vi "test Scheduled Loopback with Disable.vi"(8 "error in":errorcluster, 11 "TestCase in":refnum<class "Single Board Loopback.lvclass">) -> (0 "error out":errorcluster, 3 "TestCase out":refnum<class "Single Board Loopback.lvclass">)   [LabVIEW 2020, in "Single Board Loopback.lvclass"]
uses:
  Single Board Loopback.lvclass
  <vilib>/addons/_JKI Toolkits/VI Tester/TestCase.llb/TestCase.lvclass
  <vilib>/NI/VeriStand Custom Device Testing Tools/VeriStandTestUtilities/VeriStandTestUtilities.lvlib
  <vilib>/NI VeriStand/Execution/Workspace/NI_VS Workspace ExecutionAPI.lvlib
  <vilib>/NI VeriStand/Execution/Workspace/NI VeriStand - Set Multiple Channel Values.vi
  <vilib>/numeric/Random Number (Range) U64.vi
  C:/Program Files (x86)/National Instruments/LabVIEW 2020/vi.lib/addons/_JKI Toolkits/VI Tester/TestCase.llb/TestCase.lvclass
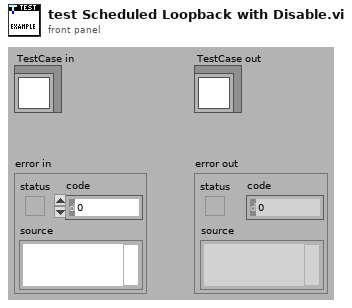
[diagram p1: front panel]
types:
  T1 = typedef "NI_VS Workspace ExecutionAPI.lvlib/WorkspaceAPI.ctl" = refnum<k24>
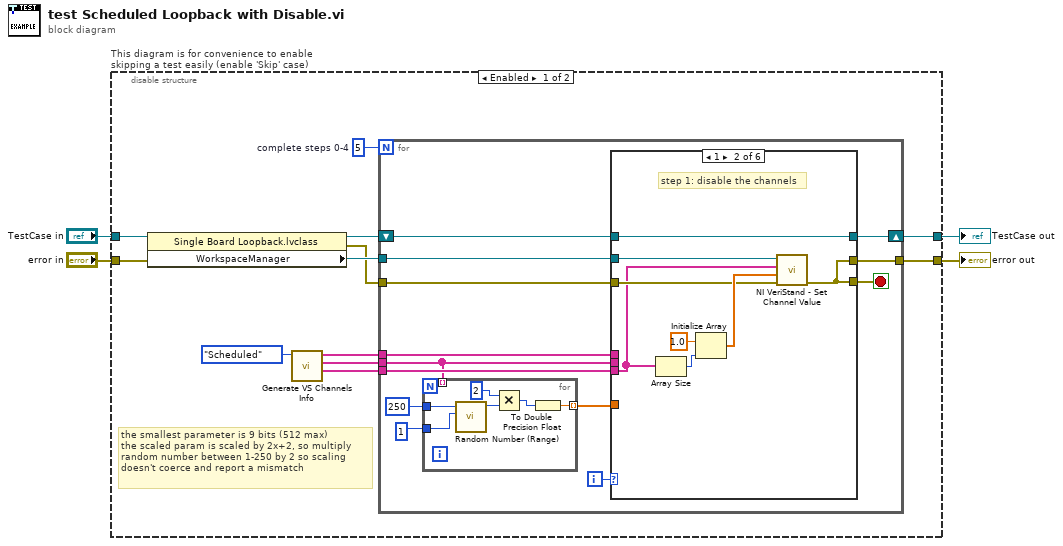
[diagram p0: block diagram]
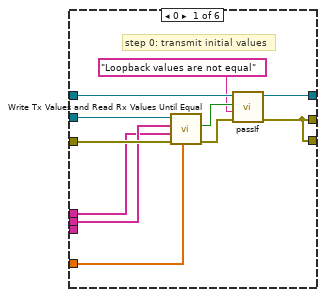
[diagram p2: hidden frame]
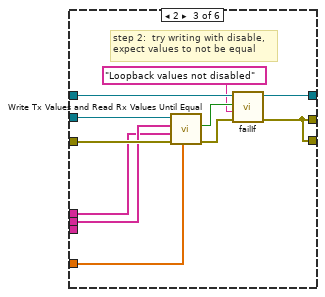
[diagram p3: hidden frame]
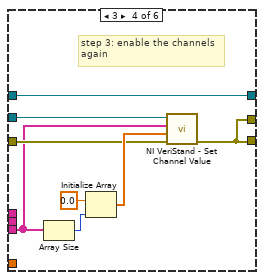
[diagram p4: hidden frame]
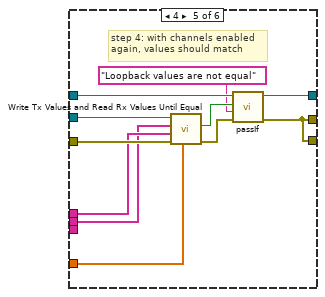
[diagram p5: hidden frame]
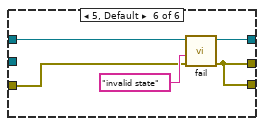
[diagram p6: hidden frame]
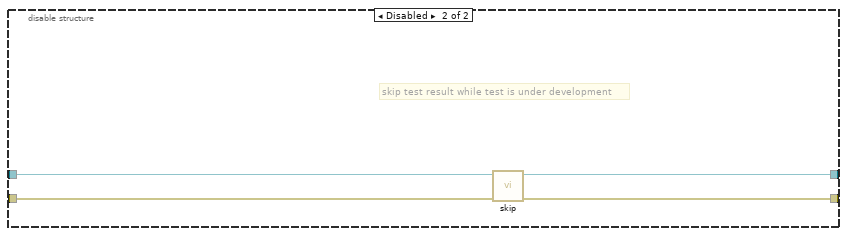
[diagram p7: hidden frame]
diagram:
  n1 = disable-structure "This diagram is for convenience to enable skipping a test easily (enable 'Skip' case)" shown="Enabled" {
    disable-tunnel: "TestCase in" -> [w12 w93]
    disable-tunnel: [w10 w91] -> w1
    disable-tunnel: [w9 w92] -> w3
    disable-tunnel: "error in" -> [w11 w90]
    frame Enabled {
      w6 = 5  # complete steps 0-4
      # "the smallest parameter is 9 bits (512 max)\nthe scaled param is scaled by 2x+2, so multiply \nrandom number between 1-250 by 2 so scaling\ndoesn't coerce and report a mismatch"
      n2 = property class="Single Board Loopback.lvclass"(reference=w12, error in=w11) -> (reference out=w13:refnum<class "Single Board Loopback.lvclass">, error out=w14:errorcluster, "WorkspaceManager"=w15:T1)
      n3 = call "Generate VS Channels Info.vi"("Transfer Type"=enum16{"Acyclic", "Scheduled"}."Scheduled") -> ("Tx Disable Channels Array"=w7:string[], "Tx Channels Array"=w8:string[], "Rx Channels Array"=w16:string[])  [unwired: 6 in, 2 out]
      n4 = for {
        N: w6 -> [_]
        tunnel: w16 -> [w29]
        tunnel: w15 -> [w28]
        tunnel: w14 -> [w27]
        tunnel: w8 -> [w17]
        shift-right: [w25] -> w10
        shift-left: w13 -> [w26]
        tunnel: [w24] -> w9
        tunnel: w7 -> [w21]
        i -> [w23]
        stop <- w22 stop-if-true
        n5 = for {
          tunnel: [w34] -> w20 mode=indexing
          tunnel: u64 250 ("upper bound (100)") -> [w33]
          tunnel: u64 1 ("upper bound (100)") -> [w32]
          tunnel: w17 -> [_] mode=indexing
          n6 = call-poly <vilib>:"Random Number (Range).vi"("lower bound (0)"=w32, "upper bound (100)"=w33) -> ("number"=w35:u64)  [unwired: 9 in]
          n7 = Multiply(x=u64 2, y=w35) -> (x*y=w31:u64)
          n8 = To Double Precision Float(number=w31) -> (double precision float=w34:dbl)
        }
        n9 = case shown="1" w23 {
          tunnel: w29 -> [w37 _ w56 _ w76 _]
          tunnel: w28 -> [w46 w50 w65 w69 w84 _]
          tunnel: w27 -> [w45 w49 w64 w68 w83 w86]
          tunnel: w26 -> [w43 w54 w62 w73 w81 w88]
          tunnel: [w42 w54 w61 w73 w80 w89] -> w25
          tunnel: [w39 w48 w58 w67 w77 w85] -> w24
          tunnel: w17 -> [w38 _ w57 _ w75 _]
          tunnel: [w39 w48 w58 w67 w77 w85] -> w22
          tunnel: w21 -> [_ w47 _ w66 _ _]
          tunnel: w20 -> [w36 _ w55 _ w74 _]
          frame 0 {
            # "step 0: transmit initial values"
            n10 = call <vilib>:"Write Tx Values and Read Rx Values Until Equal.vi"("Tx values"=w36, "error in"=w45, "Rx aliases"=w37, "Tx aliases"=w38, "workspace manager in"=w46) -> ("error out"=w44:errorcluster, "values equal"=w41:bool)  [unwired: 4 in, 1 out]
            n11 = call-dynamic "passIf.vi"("error in (no error)"=w44, "message (\"\")"="Loopback values are not equal" ("message (\"\")"), "pass"=w41, "TestCase in"=w43) -> ("error out"=w39:errorcluster, "TestCase out"=w42:refnum<class "Single Board Loopback.lvclass">)  [unwired: 6 in]
          }
          frame 1 {
            # "step 1: disable the channels"
            n12 = Array Size(array=w47) -> (size(s)=w53:i32)
            n13 = Initialize Array(1.0 ("element"), w53) -> (w51:dbl[])
            n14 = call-poly <vilib>:"NI VeriStand - Set Channel Value.vi"("error in (no error)"=w49, "Values"=w51, "Channels"=w47, "WorkspaceManager in"=w50) -> ("error out"=w48:errorcluster)  [unwired: 6 in, 1 out]
          }
          frame 2 {
            # "step 2:  try writing with disable,\nexpect values to not be equal"
            n15 = call <vilib>:"Write Tx Values and Read Rx Values Until Equal.vi"("Tx values"=w55, "error in"=w64, "Rx aliases"=w56, "Tx aliases"=w57, "workspace manager in"=w65) -> ("error out"=w63:errorcluster, "values equal"=w60:bool)  [unwired: 4 in, 1 out]
            n16 = call-dynamic "failIf.vi"("error in (no error)"=w63, "message (\"\")"="Loopback values not disabled" ("message (\"\")"), "fail"=w60, "TestCase in"=w62) -> ("error out"=w58:errorcluster, "TestCase out"=w61:refnum<class "Single Board Loopback.lvclass">)  [unwired: 6 in]
          }
          frame 3 {
            # "step 3: enable the channels\nagain"
            n17 = Array Size(array=w66) -> (size(s)=w72:i32)
            n18 = Initialize Array(0.0 ("element"), w72) -> (w70:dbl[])
            n19 = call-poly <vilib>:"NI VeriStand - Set Channel Value.vi"("error in (no error)"=w68, "Values"=w70, "Channels"=w66, "WorkspaceManager in"=w69) -> ("error out"=w67:errorcluster)  [unwired: 6 in, 1 out]
          }
          frame 4 {
            # "step 4: with channels enabled\nagain, values should match"
            n20 = call <vilib>:"Write Tx Values and Read Rx Values Until Equal.vi"("Tx values"=w74, "error in"=w83, "Rx aliases"=w76, "Tx aliases"=w75, "workspace manager in"=w84) -> ("error out"=w82:errorcluster, "values equal"=w79:bool)  [unwired: 4 in, 1 out]
            n21 = call-dynamic "passIf.vi"("error in (no error)"=w82, "message (\"\")"="Loopback values are not equal" ("message (\"\")"), "pass"=w79, "TestCase in"=w81) -> ("error out"=w77:errorcluster, "TestCase out"=w80:refnum<class "Single Board Loopback.lvclass">)  [unwired: 6 in]
          }
          frame 5, Default {
            n22 = call-dynamic "fail.vi"("error in (no error)"=w86, "message (\"\")"="invalid state" ("message (\"\")"), "TestCase in"=w88) -> ("error out"=w85:errorcluster, "TestCase out"=w89:refnum<class "Single Board Loopback.lvclass">)  [unwired: 7 in]
          }
        }
      }
    }
    frame Disabled {
      # "skip test result while test is under development"
      n23 = call <vilib>:"skip.vi"("error in (no error)"=w90, "TestCase in"=w93) -> ("error out"=w92:errorcluster, "TestCase out"=w91:refnum<class "Single Board Loopback.lvclass">)  [unwired: 8 in]
    }
  }
  "error out" <- w3
  "TestCase out" <- w1
